vi "MainHost.vi"   [LabVIEW 2018]
uses:
  Classes/Controller/User Event/User Event State.ctl
  Classes/Controller/GUI.lvclass
  Classes/IO/IO.lvclass
  Classes/S1/S1.lvclass
  Classes/Serial/Serial.lvclass
  Classes/S2/S2.lvclass
  Classes/S3/S3.lvclass
  Classes/S4/S4.lvclass
  Classes/S5/S5.lvclass
  Classes/S6/S6.lvclass
  Classes/GUI2/GUI2.lvclass
  Classes/GUI3/GUI3.lvclass
panel:
  # "LFO Test"
types:
  T1 = typedef "GUI.lvclass/User Event State.ctl" = enum16{"Create", "Get", "Destroy"}
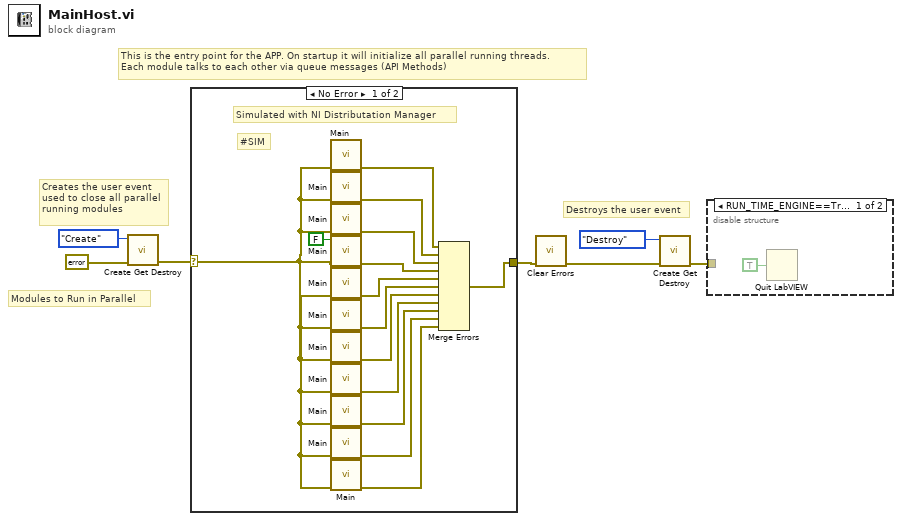
[diagram p0: block diagram]
diagram:
  # "Modules to Run in Parallel"
  # "This is the entry point for the APP. On startup it will initialize all parallel running threads. \nEach module talks to each other via queue messages (API Methods)"
  # "Destroys the user event"
  # "Creates the user event\nused to close all parallel\nrunning modules"
  n1 = call "Create Get Destroy.vi"("error In"=errorcluster {"status"=FALSE, "code"=0, "source"=""}, "State (Get)"=User_Event_State."Create") -> ("Error Out"=w3:errorcluster)  [unwired: 8 in, 1 out]
  n2 = case shown="No Error" w3 {
    selector: w3 -> [w8 w22]
    tunnel: [w21 w22] -> w7
    frame No Error {
      # "#SIM"
      # "Simulated with NI Distributation Manager"
      n3 = call "Main.vi"("error"=w8) -> ("Error out"=w11:errorcluster)  [unwired: 10 in]
      n4 = call "Main.vi"("error"=w8) -> ("Error out"=w10:errorcluster)  [unwired: 10 in]
      n5 = call "Main.vi"("error"=w8) -> ("Error out"=w9:errorcluster)  [unwired: 10 in]
      n6 = call "Main.vi"("error"=w8, "IsSimulated"=FALSE) -> ("Error out"=w20:errorcluster)  [unwired: 9 in]
      n7 = call "Main.vi"("error"=w8) -> ("Error out"=w19:errorcluster)  [unwired: 10 in]
      n8 = call "Main.vi"("error"=w8) -> ("Error out"=w18:errorcluster)  [unwired: 10 in]
      n9 = call "Main.vi"("error"=w8) -> ("Error out"=w16:errorcluster)  [unwired: 10 in]
      n10 = call "Main.vi"("error"=w8) -> ("Error out"=w15:errorcluster)  [unwired: 10 in]
      n11 = call "Main.vi"("error"=w8) -> ("Error out"=w14:errorcluster)  [unwired: 10 in]
      n12 = call "Main.vi"("error"=w8) -> ("Error out"=w13:errorcluster)  [unwired: 10 in]
      n13 = call "Main.vi"("error"=w8) -> ("Error out"=w12:errorcluster)  [unwired: 10 in]
      n14 = Merge Errors(w11, w10, w9, w20, w19, w18, w16, w15, w14, w13, w12) -> (w21:errorcluster)
    }
    frame Error {
    }
  }
  n15 = call <vilib>:"Clear Errors.vi"("error in (no error)"=w7) -> ("error out"=w6:errorcluster)  [unwired: 5 in, 1 out]
  n16 = call "Create Get Destroy.vi"("error In"=w6, "State (Get)"=User_Event_State."Destroy") -> ("Error Out"=w1:errorcluster)  [unwired: 8 in, 1 out]
  n17 = disable-structure shown="RUN_TIME_ENGINE==True" {
    disable-tunnel: w1 -> [_ _]
    frame condition #0 {
      n18 = Quit LabVIEW(quit? (T)=TRUE) -> ()
    }
    frame condition #1 (active) {
    }
  }
